vi "Time_elapsed.vi"() -> ()   [LabVIEW 2020]
panel:
  out "Elapsed Time (s)":dbl
  out "Time has Elapsed":bool
  in  "Reset":bool
  in  "Time Target (s)":dbl=15.0
  in  "stop":bool
  in  "millisecond timer value":u32
  out "RANDOM":dbl
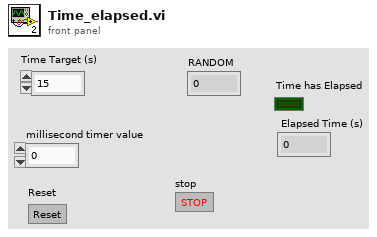
[diagram p1: front panel]
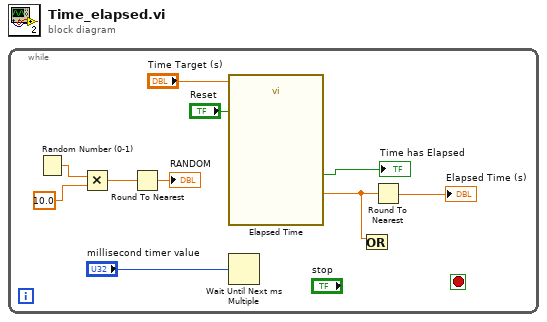
[diagram p0: block diagram]
diagram:
  n1 = while {
    stop <- _ stop-if-true
    n2 = Random Number (0-1)() -> (number: 0 to 1=w10:dbl)
    n3 = Multiply(x=w10, y=10.0 ("x*y")) -> (x*y=w2:dbl)
    n4 = Round To Nearest(number=w2) -> (nearest integer value=→"RANDOM":dbl)
    n5 = call "Elapsed Time"("Time Target (s)"="Time Target (s)", "Reset"="Reset") -> ("Elapsed Time (s)"=w1:dbl, "Time has Elapsed"=→"Time has Elapsed":bool)  [unwired: 10 in, 6 out]
    n6 = Wait Until Next ms Multiple(millisecond multiple="millisecond timer value") -> ()  [unwired: 1 out]
    n7 = Or(x=w1) -> ()  [unwired: 1 in, 1 out]
    n8 = Round To Nearest(number=w1) -> (nearest integer value=→"Elapsed Time (s)":dbl)
  }
